vi "Dashboard Main.vi"() -> ()   [LabVIEW 2018]
uses:
  Autonomous.ctl
  <vilib>/Utility/miscctls.llb/LVRowAndColumnTypeDef.ctl
  <vilib>/event_ctls.llb/eventvkey.ctl
  <vilib>/Rock Robotics/Network Tables/NT Read Boolean.vi
  <vilib>/Rock Robotics/WPI/Dashboard/WPI_DashboardLogging Global.vi
panel:
  in  "Select Auto":T1="Select Autonomous ..."
  in  "Camera Settings Right":T2={"Frame Rate"=30, "Compression"=30, "Size"=1, "DB Camera Config"=FALSE} {"Frame Rate" scale=1.0..30.0; "Compression" scale=100.0..-1.0; "Size" items=["640x480", "320x240", "160x120"]}
  in  "Camera Name Right":string(combo)="No Camera Selection"
  out "Camera Perf":string
  in  "Camera Settings":T2={"Frame Rate"=30, "Compression"=30, "Size"=1, "DB Camera Config"=FALSE} {"Frame Rate" scale=1.0..30.0; "Compression" scale=100.0..-1.0; "Size" items=["640x480", "320x240", "160x120"]}
  in  "TCP":refnum<k5>
  in  "Rec Mode":enum32{"Stop", "Record", "Playback"}(radio)
  out "Robot IP":string
  out "Image Message":string="Timeout in Camera Communications"
  in  "Dashboard Tab":T3(tab)
  out "Cargo":bool
  out "Hatch":bool
  out "NT Connection":bool
  out "Mode":T4(ring)=enum."Auto Disabled"
  out "Right Camera Perf":cluster{"Bandwidth (Mbps)":dbl, "FPS":dbl}
  in  "Auto Selector":enum16{"Airship", "Rocket"}(ring)=enum."Rocket"
  out "Camera Image Right":T5(plugin-control)
  in  "DB/String 9":string
  in  "DB/String 8":string
  in  "DB/String 7":string
  in  "DB/String 6":string
  in  "DB/String 5":string
  in  "DB/String 4":string
  in  "DB/String 3":string
  in  "DB/String 2":string
  in  "DB/String 1":string
  in  "DB/String 0":string
  in  "DB/Slider 0":dbl(slide) scale=0.0..5.0
  in  "DB/Slider 1":dbl(slide) scale=0.0..5.0
  in  "DB/Slider 2":dbl(slide) scale=0.0..5.0
  in  "DB/Slider 3":dbl(slide) scale=0.0..5.0
  out "DB/LED 3":bool
  out "DB/LED 2":bool
  out "DB/LED 1":bool
  out "DB/LED 0":bool
  in  "DB/Button 3":bool
  in  "DB/Button 2":bool
  in  "DB/Button 1":bool
  in  "DB/Button 0":bool caption="New Name"
  out "EstadoIntake":string
  out "Yaw":dbl
  out "TracaoDir":dbl
  out "TracaoEsq":dbl
  out "Elevador Position":dbl
  out "Climber Encoder":dbl
  out "Climber State":dbl
  out "Intake Position":dbl
  in  "Test Slider":dbl(slide) scale=0.0..100.0 scale format="%#_3g"
  in  "On/Off":bool caption="Solenoid"
  in  "Test Name":u16(ring) items=["Select the test to run..."]
  in  "Test Tree":string(tree)
  in  "Motor":cluster{"Value":dbl, "Enable":bool} {"Value" scale=-1.0..1.0 scale format="%#_3g"}
  out "Progress":T6 {"Test Progress" scale=0.0..100.0}
  in  "Rev/Fwd":cluster{"Forward":bool, "Reverse":bool}
  in  "Test Ring":u16(ring) items=["Monochrome", "Color"]
  out "Cmd Status":string
  in  "Execute Command":bool
  in  "Command Params":string[][](table)
  in  "Command Selection":i32(listbox)
  in  "CheckList":i32(listbox)
  out "Tree":string(tree)
  out "Camera Image":T5(plugin-control)
  out "Background":bool
  in  "Camera Name":string(combo)="No Camera Selection"
  # "HW"
  # "HW"
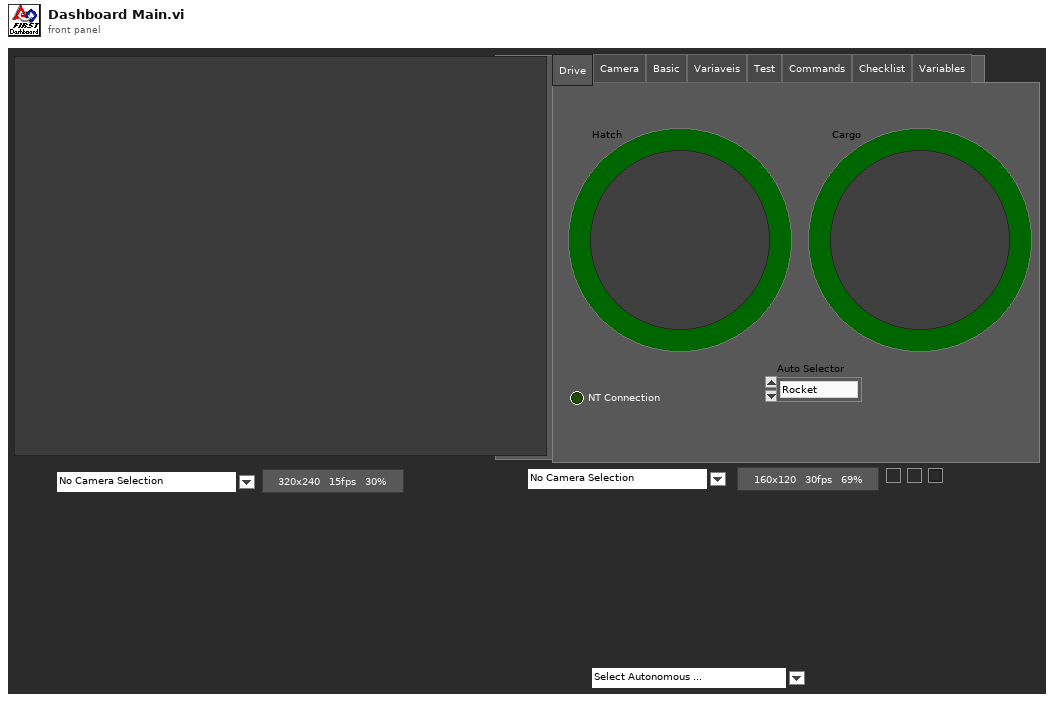
[diagram p1: front panel]
types:
  T1 = typedef "Autonomous.ctl" = string
  T2 = cluster{"Frame Rate":i32, "Compression":i32, "Size":u16, "DB Camera Config":bool}
  T3 = enum32{"Drive", "Camera", "Basic", "Variaveis", "Test", "Commands", "Checklist", "Variables"}
  T4 = enum8{"Tele-Op Disabled", "Tele-Op Enabled", "Auto Disabled", "Auto Enabled", "Test Disabled", "Test Enabled", "Disconnected", "No Code", "E-Stop"}
  T5 = typedef "IMAQ Image.ctl" = refnum<image>
  T6 = cluster{"Test Progress":u8, "Test Progress Text":string}
  T7 = cluster{"Save Path":path, "Interval (s)":dbl, "Keep":i32}
  T8 = enum32{"Drive", "Camera", "Basic", "Custom", "Test", "Commands", "Checklist", "Variables"}
  T9 = typedef "Image Type" = u32
  T10 = cluster{"IDs":cluster{"RPC field ID":u16, "Unique ID":u16}, "String":string}
  T11 = cluster{"Error Strings":string, "Disable Counts":cluster{u16, u16}, "Rail Faults":cluster{u16, u16, u16}, "Robot IP":string, "DB Mode":u8, "Event Info":cluster{"Name":string, "Type":u8, "Number":u16, "Replay":u8}}
  T12 = cluster{"Storage":cluster{"Disk Free":u64, "RAM Block":u32, "RAM free":u32}, "CPU Utilization":cluster{"CPU % ISR":sgl, "CPU % Time Crit":sgl, "CPU % Timed Str":sgl, "CPU % High":sgl, "CPU % Above":sgl, "CPU % Normal":sgl, "CPU % Low":sgl}, "CAN":cluster{"% Bus Utilization":sgl, "Bus Off Cnt":u32, "TX_FIFO Full Cnt":u32, "Receive Error Cnt":u8, "Transmit Error Cnt":u8}, "HID":cluster{"HID Outputs":u32, "Rumble Low":u16, "Rumble High":u16}[]}
  T13 = cluster{"Status bits":cluster{"Test Mode":bool, "Autonomous":bool, "Enabled":bool, "Code Start":bool, "Brownout":bool, "Reserved 2":bool, "Reserved 3":bool, "E-Stop":bool}, "Code Trace":cluster{"Disabled":bool, "TeleOp":bool, "Auto":bool, "Test":bool}, "Controller Type":enum16{"unknown", "cRIO", "roboRio"}, "Code?":enum16{"unknown", "noCode", "code"}, "Battery V":dbl}
  T14 = cluster{"Control Bits":cluster{"TestMode":bool, "Autonomous":bool, "Enabled":bool, "FMS Present":bool, bool, bool, bool, "E-Stop":bool}, "Team Station ":u8, "Countdown":sgl, "Joystick Values":cluster{"Axes":dbl[], "Buttons":bool[], "POVs":i16[]}[]}
  T15 = cluster{"Camera Image":refnum<vi>, "Dashboard Tab":refnum<vi>, "Background":refnum<vi>, "Rec Mode":refnum<vi>, "Test Slider":refnum<vi>, "On/Off ":refnum<vi>, "Test Ring":refnum<vi>, "Rev/Fwd":refnum<vi>, "Test Name":refnum<vi>, "Motor":refnum<vi>, "Progress":refnum<vi>, "CheckList":refnum<vi>, "Tree":refnum<vi>, "Test Tree":refnum<vi>, "Command Params":refnum<vi>, "Command Selection":refnum<vi>, "Execute Command":refnum<vi>, "Cmd Status":refnum<vi>, "Camera Settings":refnum<vi>, "Camera Name":refnum<vi>, "Camera Perf":refnum<vi>, "Camera Settings Right":refnum<vi>, "Camera Name Right":refnum<vi>, "Camera Image Right":refnum<vi>}
  T16 = cluster{"Global Rectangle":i32[], "Contours":cluster{"Contour Type":u32, "ROI Type":u32, "Points":i32[]}[]}
  T17 = cluster{"Camera Name":string, string, "Saved DB Images Info":cluster{"Save Path":path, "Interval (s)":dbl, "Keep":i32}}
  T18 = cluster{"Camera Name Right":string, string, "Saved DB Images Info":cluster{"Save Path":path, "Interval (s)":dbl, "Keep":i32}}
  T19 = cluster{"Operation":enum16{"Update", "Clear"}, "Color Box":u32}[]
  T20 = typedef "eventvkey.ctl" = enum16{"ASCII", "Enter", "Return", "Shift", "Ctrl", "Alt", "Cmd", "Opt", "Caps", "NumLock", "Clear", "Break", "Up", "Down", "Left", "Right", "Insert", "Delete", "Home", "End", "PageUp", "PageDown", "Escape", "Help", "Pause", "ScrollLock", "F1", "F2", "F3", "F4", "F5", "F6", "F7", "F8", "F9", "F10", "F11", "F12", "F13", "F14", "F15", "F16", "F17", "F18", "F19", "F20", "F21", "F22", "F23", "F24", "Play", "VolumeUp", "VolumeDown", "Mute", "Two Byte Char"}
  T21 = cluster{"Image Size":bool, "Image Type":bool, "Pixel Value":bool, "ROI Information":bool, "Zoom Factor":bool}
  T22 = cluster{"Operation":enum16{"Update", "Clear"}, "Color Box":u32}
  T23 = typedef "LVRowAndColumnTypeDef.ctl" = cluster{"Row":i32, "Column":i32}
  T24 = cluster{"Shift":bool, "Ctrl":bool, "Alt":bool, "Cmd":bool, "Opt":bool}
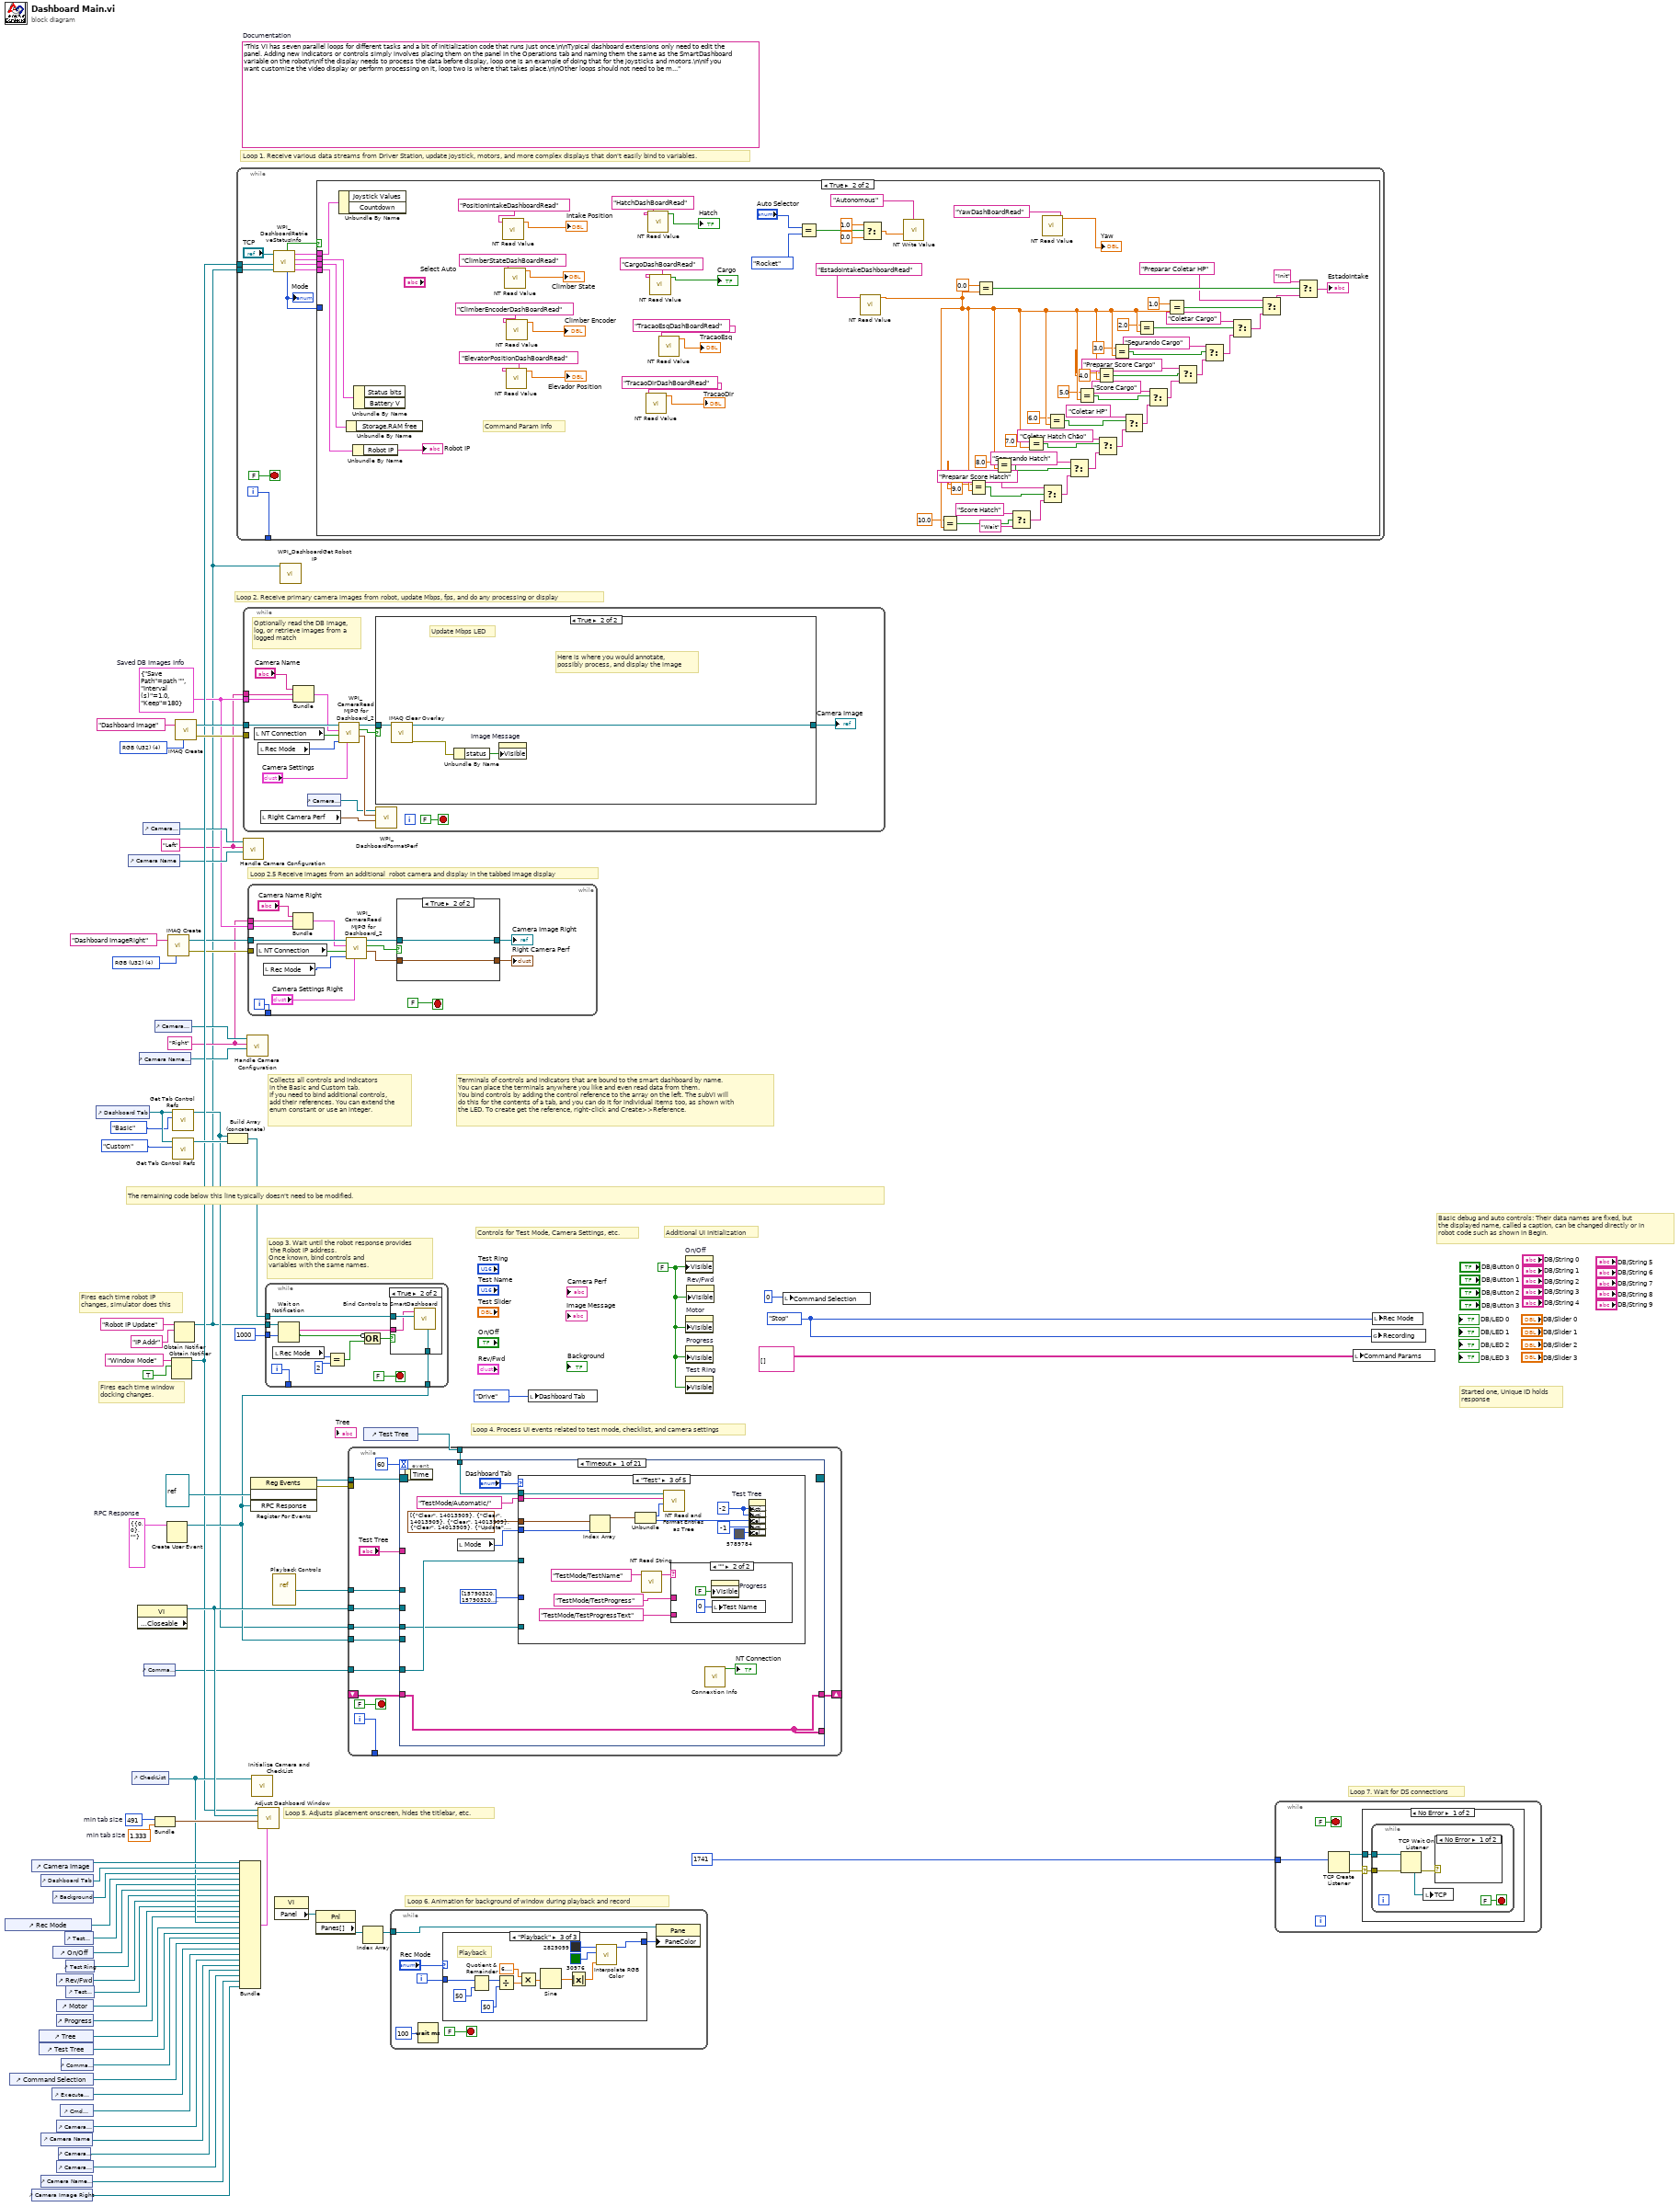
[diagram p0: block diagram]
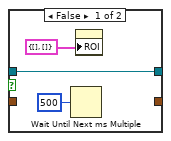
[diagram p2: hidden frame]
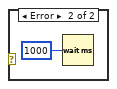
[diagram p3: hidden frame]
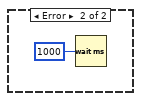
[diagram p4: hidden frame]
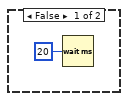
[diagram p5: hidden frame]
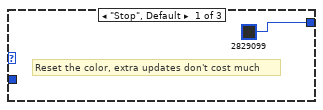
[diagram p6: hidden frame]
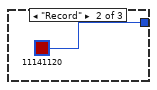
[diagram p7: hidden frame]
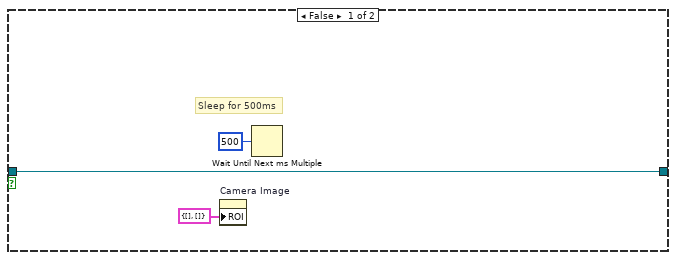
[diagram p9: hidden frame]
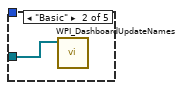
[diagram p11: hidden frame]
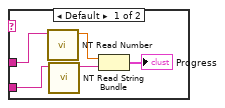
[diagram p12: hidden frame]
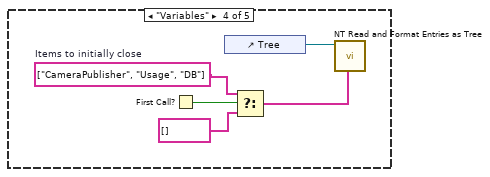
[diagram p13: hidden frame]
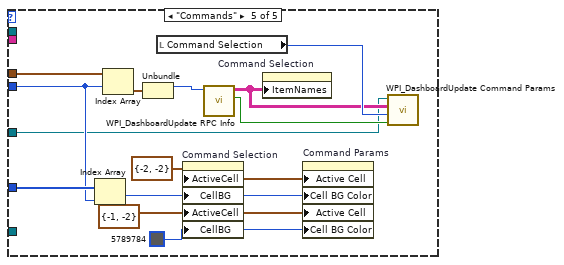
[diagram p14: hidden frame]
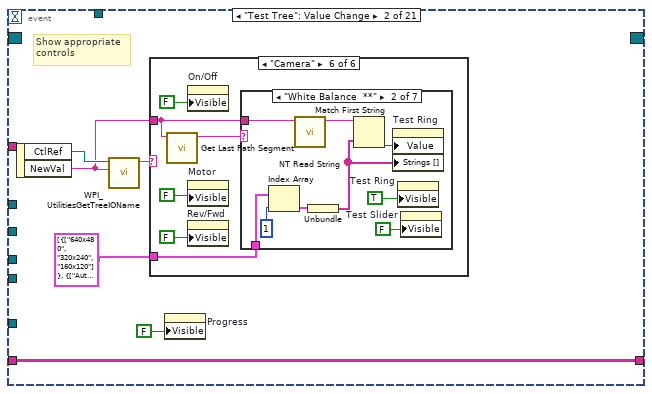
[diagram p15: hidden frame]
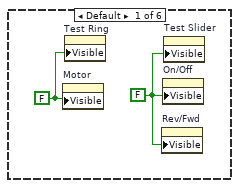
[diagram p16: hidden frame]
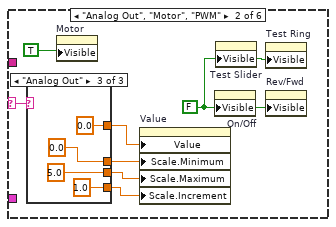
[diagram p17: hidden frame]
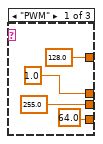
[diagram p18: hidden frame]
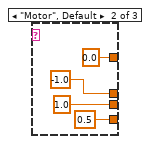
[diagram p19: hidden frame]
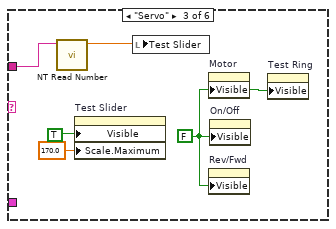
[diagram p20: hidden frame]
diagram:
  w4 = T7 {"Save Path"=path "", "Interval (s)"=1.0, "Keep"=180}  # Saved DB Images Info
  w3 = "Right"
  w2 = "Left"
  w14 = T9 4 items=["Grayscale (U8)", "Grayscale (I16)", "Grayscale (SGL)", "Complex (CSG)", "RGB (U32)", "HSL (U32)", "RGB (U64)"] ("Image Type")
  w28 = T10 {"IDs"={"RPC field ID"=0, "Unique ID"=0}, "String"=""}  # RPC Response
  w50 = 491  # min tab size
  w49 = 1.333  # min tab size
  w57 = enum32{"Stop", "Record", "Playback"}."Stop" ("Rec Mode")
  w34 = FALSE ("Visible")
  (unwired) "This VI has seven parallel loops for different tasks and a bit of initialization code that runs just once.\n\nTypical dashboard extensions only need to edit the panel. Adding new indicators or controls simply involves placing them on the panel in the Operations tab and naming them the same as the SmartDashboard variable on the robot\n\nIf the display needs to process the data before display, loop one is an example of doing that for the joysticks and motors.\n\nIf you want customize the video display or perform processing on it, loop two is where that takes place.\n\nOther loops should not need to be modified. They are pretty standard, and document the task they perform."  # Documentation
  w74 = T9 4 items=["Grayscale (U8)", "Grayscale (I16)", "Grayscale (SGL)", "Complex (CSG)", "RGB (U32)", "HSL (U32)", "RGB (U64)"] ("Image Type")
  # "Loop 2.5 Receive images from an additional  robot camera and display in the tabbed image display"
  # "Started one, Unique ID holds\nresponse"
  # "Loop 7. Wait for DS connections"
  # "Basic debug and auto controls: Their data names are fixed, but\nthe displayed name, called a caption, can be changed directly or in\nrobot code such as shown in Begin."
  # "Controls for Test Mode, Camera Settings, etc."
  # "Additional UI Initialization"
  # "Loop 6. Animation for background of window during playback and record"
  # "Fires each time robot IP\nchanges, simulator does this"
  # "Fires each time window\ndocking changes."
  # "Collects all controls and indicators\nin the Basic and Custom tab.\nIf you need to bind additional controls,\nadd their references. You can extend the\nenum constant or use an integer."
  # "The remaining code below this line typically doesn't need to be modified."
  # "Loop 4. Process UI events related to test mode, checklist, and camera settings"
  # "Terminals of controls and indicators that are bound to the smart dashboard by name.\nYou can place the terminals anywhere you like and even read data from them.\nYou bind controls by adding the control reference to the array on the left. The subVI will\ndo this for the contents of a tab, and you can do it for individual items too, as shown with\nthe LED. To create get the reference, right-click and Create>>Reference."
  # "Loop 3. Wait until the robot response provides\n the Robot IP address.\nOnce known, bind controls and\nvariables with the same names."
  # "Loop 5. Adjusts placement onscreen, hides the titlebar, etc."
  # "Loop 1. Receive various data streams from Driver Station, update joystick, motors, and more complex displays that don't easily bind to variables."
  # "Loop 2. Receive primary camera images from robot, update Mbps, fps, and do any processing or display"
  n1 = control-ref of="Rec Mode"() -> (w40:refnum<vi>)
  n2 = control-ref of="Command Selection"() -> (w27:refnum<vi>)
  n3 = control-ref of="Camera Image Right"() -> (w7:refnum<vi>)
  n4 = control-ref of="Camera Image"() -> (w52:refnum<vi>)
  n5 = control-ref of="Tree"() -> (w44:refnum<vi>)
  n6 = control-ref of="Test Tree"() -> (w43:refnum<vi>)
  n7 = control-ref of="Dashboard Tab"() -> (w51:refnum<vi>)
  n8 = control-ref of="Camera Name"() -> (w18:refnum<vi>)
  n9 = control-ref of="Camera Name Right"() -> (w8:refnum<vi>)
  n10 = control-ref of="Execute Command"() -> (w29:refnum<vi>)
  n11 = control-ref of="Background"() -> (w47:refnum<vi>)
  n12 = control-ref of="On/Off"() -> (w38:refnum<vi>)
  n13 = control-ref of="Progress"() -> (w35:refnum<vi>)
  n14 = control-ref of="Camera Settings"() -> (w19:refnum<vi>)
  n15 = control-ref of="Camera Settings Right"() -> (w9:refnum<vi>)
  n16 = control-ref of="Rev/Fwd"() -> (w36:refnum<vi>)
  n17 = control-ref of="Motor"() -> (w41:refnum<vi>)
  n18 = control-ref of="Camera Perf"() -> (w17:refnum<vi>)
  n19 = control-ref of="Cmd Status"() -> (w23:refnum<vi>)
  n20 = control-ref of="Command Params"() -> (w30:refnum<vi>)
  n21 = control-ref of="Test Slider"() -> (w39:refnum<vi>)
  n22 = control-ref of="Test Ring"() -> (w37:refnum<vi>)
  n23 = control-ref of="Test Name"() -> (w42:refnum<vi>)
  n24 = control-ref of="Dashboard Tab"() -> (w55:refnum<vi>)
  n25 = control-ref of="Camera Name"() -> (w20:refnum<vi>)
  n26 = control-ref of="CheckList"() -> (w45:refnum<vi>)
  n27 = property class="VI" props=["Front Panel.Closeable"]() -> (reference out=w56:refnum<vi>)  [unwired: 2 in, 2 out]
  n28 = control-ref of="Camera Name Right"() -> (w10:refnum<vi>)
  n29 = control-ref of="Camera Settings"() -> (w21:refnum<vi>)
  n30 = control-ref of="Command Params"() -> (w22:refnum<vi>)
  n31 = control-ref of="Camera Settings Right"() -> (w11:refnum<vi>)
  n32 = Bundle("min tab size"=w50, "min tab size"=w49) -> (w48:cluster{"min tab size":i32, "min tab size":dbl})  [unwired: 1 in]
  n33 = Create User Event(user event datatype=w28) -> (user event=w24:refnum<user-event>)  [unwired: 1 in, 1 out]
  n34 = call "IMAQ Create"("Image Name"="Dashboard ImageRight", "Image Type"=w14) -> ("New Image"=w13:T5, "error out"=w12:errorcluster)  [unwired: 2 in, 1 out]
  n35 = Obtain Notifier(name (unnamed)="Window Mode", notification data type=TRUE) -> (notifier out=w33:refnum<notifier>)  [unwired: 2 in, 2 out]
  n36 = call <vilib>:"Get Tab Control Refs.vi"("Page Index"=T8."Basic" ("Dashboard Tab"), "TabControl in"=w55) -> ("ControlsOnPage"=w16:refnum<vi>[])  [unwired: 9 in]
  n37 = call <vilib>:"Get Tab Control Refs.vi"("Page Index"=T8."Custom" ("Dashboard Tab"), "TabControl in"=w55) -> ("ControlsOnPage"=w54:refnum<vi>[])  [unwired: 9 in]
  n38 = Obtain Notifier(name (unnamed)="Robot IP Update", notification data type="IP Addr" ("name (unnamed)")) -> (notifier out=w1:refnum<notifier>)  [unwired: 2 in, 2 out]
  n39 = call "IMAQ Create"("Image Name"="Dashboard Image", "Image Type"=w74) -> ("New Image"=w72:T5, "error out"=w71:errorcluster)  [unwired: 2 in, 1 out]
  n40 = Build Array (concatenate)(w16, w54) -> (w53:refnum<vi>[])
  n41 = while {
    tunnel: [w84] -> _
    tunnel: w1 -> [w78]
    tunnel: w33 -> [w75]
    i -> [w84]
    stop <- FALSE stop-if-true
    n42 = call <vilib>:"WPI_DashboardRetrieveStatusInfo.vi"("Binding Refnum"=w78, "Window Mode Notifier"=w75, "TCP Cnx"="TCP") -> ("Power and Errors"=w79:T11, "Robot Metrics"=w82:T12, "Status Info"=w83:T13, "Control Info"=w80:T14, "Robot Mode"=w77:T4, "Process?"=w81:bool)  [unwired: 3 in]
    "Mode" <- w77
    n43 = case shown="True" w81 {
      tunnel: w83 -> [_ w163]
      tunnel: w82 -> [_ w162]
      tunnel: w80 -> [_ w161]
      tunnel: w79 -> [_ w160]
      tunnel: w77 -> [_ _]
      frame False {
        n44 = Wait (ms)(milliseconds to wait=u32 20) -> ()  [unwired: 1 out]
      }
      frame True {
        # "Command Param Info"
        n45 = Unbundle By Name(w161) -> ()  [unwired: 2 out]
        n46 = Unbundle By Name(w162) -> ()  [unwired: 1 out]
        n47 = Unbundle By Name(w160) -> ("Robot IP"=→"Robot IP":string)
        n48 = Unbundle By Name(w163) -> ()  [unwired: 2 out]
        n49 = call-poly <vilib>:"NT Read Value.vi"("Name"="PositionIntakeDashboardRead") -> ("Numeric"=→"Intake Position":dbl)  [unwired: 9 in, 1 out]
        n50 = call-poly <vilib>:"NT Read Value.vi"("Name"="ClimberStateDashBoardRead") -> ("Numeric"=→"Climber State":dbl)  [unwired: 9 in, 1 out]
        n51 = call-poly <vilib>:"NT Read Value.vi"("Name"="ElevatorPositionDashBoardRead") -> ("Numeric"=→"Elevador Position":dbl)  [unwired: 9 in, 1 out]
        n52 = call-poly <vilib>:"NT Read Value.vi"("Name"="ClimberEncoderDashBoardRead") -> ("Numeric"=→"Climber Encoder":dbl)  [unwired: 9 in, 1 out]
        n53 = call-poly <vilib>:"NT Read Value.vi"("Name"="TracaoDirDashBoardRead") -> ("Numeric"=→"TracaoDir":dbl)  [unwired: 9 in, 1 out]
        n54 = call-poly <vilib>:"NT Read Value.vi"("Name"="HatchDashBoardRead") -> ("Boolean"=→"Hatch":bool)  [unwired: 9 in, 1 out]
        n55 = call-poly <vilib>:"NT Read Value.vi"("Name"="CargoDashBoardRead") -> ("Boolean"=→"Cargo":bool)  [unwired: 9 in, 1 out]
        n56 = call-poly <vilib>:"NT Read Value.vi"("Name"="TracaoEsqDashBoardRead") -> ("Numeric"=→"TracaoEsq":dbl)  [unwired: 9 in, 1 out]
        n57 = Equal?(x="Auto Selector", y=enum16{"Airship", "Rocket"}."Rocket") -> (x = y?=w141:bool)
        n58 = call-poly <vilib>:"NT Read Value.vi"("Name"="EstadoIntakeDashboardRead") -> ("Numeric"=w135:dbl)  [unwired: 9 in, 1 out]
        n59 = Select(t=1.0, s=w141, f=0.0) -> (s? t:f=w142:dbl)
        n60 = call-poly <vilib>:"NT Write Value.vi"("Numeric"=w142, "Name"="Autonomous") -> ()  [unwired: 9 in, 1 out]
        n61 = Equal?(x=10.0, y=w135) -> (x = y?=w134:bool)
        n62 = Equal?(x=9.0, y=w135) -> (x = y?=w133:bool)
        n63 = Equal?(x=0.0, y=w135) -> (x = y?=w113:bool)
        n64 = Equal?(x=8.0, y=w135) -> (x = y?=w132:bool)
        n65 = Select(t="Score Hatch", s=w134, f="Wait") -> (s? t:f=w126:string)
        n66 = Equal?(x=7.0, y=w135) -> (x = y?=w131:bool)
        n67 = call-poly <vilib>:"NT Read Value.vi"("Name"="YawDashBoardRead") -> ("Numeric"=→"Yaw":dbl)  [unwired: 9 in, 1 out]
        n68 = Select(t="Preparar Score Hatch", s=w133, f=w126) -> (s? t:f=w125:string)
        n69 = Equal?(x=6.0, y=w135) -> (x = y?=w130:bool)
        n70 = Select(t="Segurando Hatch", s=w132, f=w125) -> (s? t:f=w124:string)
        n71 = Equal?(x=5.0, y=w135) -> (x = y?=w129:bool)
        n72 = Equal?(x=4.0, y=w135) -> (x = y?=w128:bool)
        n73 = Select(t="Coletar Hatch Chão", s=w131, f=w124) -> (s? t:f=w123:string)
        n74 = Equal?(x=3.0, y=w135) -> (x = y?=w127:bool)
        n75 = Select(t="Coletar HP", s=w130, f=w123) -> (s? t:f=w122:string)
        n76 = Equal?(x=2.0, y=w135) -> (x = y?=w117:bool)
        n77 = Select(t="Score Cargo", s=w129, f=w122) -> (s? t:f=w121:string)
        n78 = Equal?(x=1.0, y=w135) -> (x = y?=w116:bool)
        n79 = Select(t="Preparar Score Cargo", s=w128, f=w121) -> (s? t:f=w120:string)
        n80 = Select(t="Segurando Cargo", s=w127, f=w120) -> (s? t:f=w119:string)
        n81 = Select(t="Coletar Cargo", s=w117, f=w119) -> (s? t:f=w118:string)
        n82 = Select(t="Preparar Coletar HP", s=w116, f=w118) -> (s? t:f=w115:string)
        n83 = Select(t="Init", s=w113, f=w115) -> (s? t:f=→"EstadoIntake":string)
      }
    }
  }
  n84 = Bundle("Camera Image"=w52, "Dashboard Tab"=w51, "Background"=w47, "Rec Mode"=w40, "Test Slider"=w39, "On/Off"=w38, "Test Ring"=w37, "Rev/Fwd"=w36, "Test Name"=w42, "Motor"=w41, "Progress"=w35, "CheckList"=w45, "Tree"=w44, "Test Tree"=w43, "Command Params"=w30, "Command Selection"=w27, "Execute Command"=w29, "Cmd Status"=w23, "Camera Settings"=w19, "Camera Name"=w18, "Camera Perf"=w17, "Camera Settings Right"=w9, "Camera Name Right"=w8, "Camera Image Right"=w7) -> (w46:T15)  [unwired: 1 in]
  n85 = call "Handle Camera Configuration.vi"("CameraNameRef"=w20, "Display Name"=w2, "ClusterRef"=w21) -> ()  [unwired: 9 in]
  n86 = while {
    tunnel: w72 -> [w177]
    tunnel: w71 -> [_]
    tunnel: w4 -> [w170]
    tunnel: w2 -> [w167]
    stop <- FALSE stop-if-true
    # "Optionally read the DB image,\nlog, or retrieve images from a\nlogged match"
    n87 = local read "NT Connection"() -> (w171:bool)
    n88 = local read "Rec Mode"() -> (w174:enum32{"Stop", "Record", "Playback"})
    n89 = local read "Right Camera Perf"() -> (w165:cluster{"Bandwidth (Mbps)":dbl, "FPS":dbl})
    n90 = Bundle("Camera Name"="Camera Name", w167, "Saved DB Images Info"=w170) -> (w169:T17)  [unwired: 1 in]
    n91 = control-ref of="Camera Perf"() -> (w164:refnum<vi>)
    n92 = call <vilib>:"WPI_CameraRead MJPG for Dashboard_2.vi"("Camera Settings"="Camera Settings", "Rec Mode"=w174, "NT Connection"=w171, "Capture Info"=w169, "Image in"=w177) -> ("perf info"=w166:cluster{"Bandwidth (Mbps)":dbl, "fps":dbl}, "Active"=w175:bool, "Image\\ out"=w176:T5)  [unwired: 4 in]
    n93 = case shown="True" w175 {
      tunnel: w176 -> [w180 w183]
      tunnel: [w180 w182] -> w172
      frame False {
        # "Sleep for 500ms"
        n94 = property on="Camera Image" class="ImageControl"("ROI"=T16 {"Global Rectangle"=[], "Contours"=[]}) -> ()  [unwired: 2 in, 2 out]
        n95 = Wait Until Next ms Multiple(millisecond multiple=u32 500) -> ()  [unwired: 1 out]
      }
      frame True {
        # "Here is where you would annotate,\npossibly process, and display the image"
        # "Update Mbps LED"
        n96 = call "IMAQ Clear Overlay"("Image"=w183) -> ("error out"=w184:errorcluster, "Image Out"=w182:T5)  [unwired: 2 in, 7 out]
        n97 = Unbundle By Name(w184) -> ("status"=w185:bool)
        n98 = property on="Image Message" class="Str"("Visible"=w185) -> ()  [unwired: 2 in, 2 out]
      }
    }
    "Camera Image" <- w172
    n99 = call <vilib>:"WPI_DashboardFormatPerf.vi"("Right Camera Perf"=w165, "Performance"=w166, "String in"=w164) -> ()  [unwired: 9 in]
  }
  n100 = call "Handle Camera Configuration.vi"("CameraNameRef"=w10, "Display Name"=w3, "ClusterRef"=w11) -> ()  [unwired: 9 in]
  n101 = while {
    tunnel: w13 -> [w200]
    tunnel: w12 -> [_]
    tunnel: [w195] -> _
    tunnel: w4 -> [w191]
    tunnel: w3 -> [w188]
    i -> [w195]
    stop <- FALSE stop-if-true
    n102 = local read "NT Connection"() -> (w192:bool)
    n103 = local read "Rec Mode"() -> (w199:enum32{"Stop", "Record", "Playback"})
    n104 = Bundle("Camera Name Right"="Camera Name Right", w188, "Saved DB Images Info"=w191) -> (w190:T18)  [unwired: 1 in]
    n105 = call <vilib>:"WPI_CameraRead MJPG for Dashboard_2.vi"("Camera Settings"="Camera Settings Right", "Rec Mode"=w199, "NT Connection"=w192, "Capture Info"=w190, "Image in"=w200) -> ("perf info"=w186:cluster{"Bandwidth (Mbps)":dbl, "fps":dbl}, "Active"=w194:bool, "Image\\ out"=w197:T5)  [unwired: 4 in]
    n106 = case shown="True" w194 {
      tunnel: w197 -> [w202 w205]
      tunnel: [w202 w205] -> w193
      tunnel: [_ w204] -> w187
      tunnel: w186 -> [_ w204]
      frame False {
        n107 = Wait Until Next ms Multiple(millisecond multiple=u32 500) -> ()  [unwired: 1 out]
        n108 = property on="Camera Image Right" class="ImageControl"("ROI"=T16 {"Global Rectangle"=[], "Contours"=[]}) -> ()  [unwired: 2 in, 2 out]
      }
      frame True {
      }
    }
    "Camera Image Right" <- w193
    "Right Camera Perf" <- w187
  }
  n109 = register-events(refnum<vi> refnum, w24) -> (reference out=w61:refnum<event-registration>, error out=w60:errorcluster)  [unwired: 2 in]
  n110 = call "Initialize Camera and CheckList.vi"("ListBox in"=w45) -> ()  [unwired: 11 in]
  n111 = call "Adjust Dashboard Window.vi"("Sizing Refnums"=w46, "Size Constraints"=w48, "VI"=w56, "WIn Mode"=w33) -> ()  [unwired: 8 in]
  n112 = while {
    tunnel: w53 -> [w217]
    tunnel: w1 -> [w215]
    tunnel: [w213] -> _
    tunnel: u32 1000 ("milliseconds to wait") -> [w212]
    tunnel: w24 -> [w206]
    i -> [w213]
    stop <- FALSE stop-if-true
    n113 = local read "Rec Mode"() -> (w208:enum32{"Stop", "Record", "Playback"})
    n114 = Wait on Notification(notifier=w215, timeout in ms (-1)=w212) -> (notification=w214:string, timed out?=w210:bool)  [unwired: 2 in, 2 out]
    n115 = Equal?(x=w208, y=u16 2 ("Rec Mode")) -> (x = y?=w209:bool)
    n116 = Compound Arithmetic op=OR(invert w210, w209) -> (w211:bool)
    n117 = case shown="True" w211 {
      tunnel: w217 -> [_ w220]
      tunnel: w214 -> [_ w219]
      tunnel: w206 -> [_ w218]
      frame False {
      }
      frame True {
        n118 = call <vilib>:"Bind Controls to SmartDashboard.vi"("RPC ref"=w218, "Bound Control Refs"=w220, "Server IP Address"=w219) -> ()  [unwired: 9 in]
      }
    }
  }
  n119 = vi-ref "Playback Controls.vi"() -> (w62:refnum<vi>)
  n120 = property class="VI"() -> ("Panel"=w64:refnum<vi>)  [unwired: 2 in, 2 out]
  n121 = call "WPI_DashboardGet Robot IP.vi"("Notifier in"=w1) -> ()  [unwired: 11 in]
  n122 = property class="Pnl"(reference=w64) -> ("Panes[]"=w65:refnum<vi>[])  [unwired: 1 in, 2 out]
  n123 = Index Array(array=w65) -> (element=w63:refnum<vi>)  [unwired: 1 in]
  n124 = control-ref of="Test Tree"() -> (w66:refnum<vi>)
  n125 = while {
    tunnel: [w230] -> _
    tunnel: w66 -> [w229]
    tunnel: w62 -> [w228]
    tunnel: w61 -> [w227]
    tunnel: w60 -> [_]
    tunnel: w56 -> [w226]
    tunnel: w24 -> [w225]
    tunnel: w22 -> [w224]
    shift-right: [w223] -> _
    shift-left: _ -> [w222]
    tunnel: w16 -> [w221]
    i -> [w230]
    stop <- FALSE stop-if-true
    n126 = event shown="[0] Timeout" {
      selector: w227 -> [_ _ _ _ _ _ _ _ _ _ _ _ _ _ _ _ _ _ _ _ _]
      dyn-events: [_ _ _ _ _ _ _ _ _ _ _ _ _ _ _ _ w490 _ _ _ _] -> _
      timeout: u32 60 ("milliseconds to wait") -> [_ _ _ _ _ _ _ _ _ _ _ _ _ _ _ _ _ _ _ _ _]
      tunnel: w229 -> [w242 _ _ _ _ _ _ _ _ _ _ _ _ _ _ _ _ _ _ _ _]
      tunnel: "Test Tree" -> [_ _ _ _ _ _ _ _ _ _ _ w457 w465 w467 w471 w479 _ _ _ _ _]
      tunnel: w228 -> [_ _ _ _ _ _ _ _ _ _ _ _ _ _ _ _ w492 _ w510 _ _]
      tunnel: w226 -> [_ _ _ _ _ _ _ _ _ _ _ _ _ _ _ _ w488 _ _ _ _]
      tunnel: w225 -> [_ _ _ _ _ _ _ _ _ _ _ _ _ _ _ _ w486 _ _ _ _]
      tunnel: w224 -> [w237 _ _ _ _ _ w408 _ _ _ _ _ _ _ _ _ _ _ _ _ _]
      tunnel: [w234 w285 w387 w392 w401 w405 w406 w415 w425 w432 w444 w456 w463 w466 w470 w478 w485 w505 w507 w511 w524] -> w223
      tunnel: w222 -> [w234 w285 w387 w392 w401 w405 w406 _ _ w432 w444 w456 w463 w466 w470 w478 w485 w505 w507 w511 w524]
      tunnel: w221 -> [w235 _ _ _ _ _ _ _ _ _ _ _ _ _ _ _ _ _ _ _ _]
      tunnel: [w234 _ _ _ _ _ _ _ _ _ _ _ _ _ _ _ _ _ _ _ _] -> _
      event Timeout {
        n127 = event-data() -> ()  [unwired: 1 in, 1 out]
        n128 = local read "Mode"() -> (w239:T4)
        n129 = case shown="\"Test\"" "Dashboard Tab" {
          tunnel: w242 -> [_ _ w258 _ _]
          tunnel: "TestMode/Automatic/" ("Name Pattern") -> [_ _ w257 _ _]
          tunnel: T19 [{"Operation"=enum."Clear", "Color Box"=14013909}, {"Operation"=enum."Clear", "Color Box"=14013909}, {"Operation"=enum."Clear", "Color Box"=14013909}, {"Operation"=enum."Clear", "Color Box"=14013909}, {"Operation"=enum."Update", "Color Box"=14013909}, {"Operation"=enum."Update", "Color Box"=16777215}, {"Operation"=enum."Clear", "Color Box"=14013909}, {"Operation"=enum."Clear", "Color Box"=14013909}, {"Operation"=enum."Clear", "Color Box"=14013909}] -> [_ _ w250 _ w278]
          tunnel: w239 -> [_ _ w249 _ w277]
          tunnel: u32[] [15790320, 15790320, 15790320, 15790320, 16777215, 16777215, 15790320, 15790320, 15790320] -> [_ _ _ _ w283]
          tunnel: w237 -> [_ _ _ _ w271]
          tunnel: w235 -> [_ w244 _ _ _]
          frame "Variaveis", Default {
          }
          frame "Basic" {
            n130 = call <vilib>:"WPI_DashboardUpdateNames.vi"("Controls on Tab"=w244) -> ()  [unwired: 11 in]
          }
          frame "Test" {
            w256 = -2 ("Active Item:Row Number")
            n131 = Index Array(array=w250, index=w249) -> (element=w251:T22)
            n132 = Unbundle(w251) -> ("Operation"=w252:enum16{"Update", "Clear"}, "Color Box"=w253:u32)
            n133 = call <vilib>:"NT Read String.vi"("Name"="TestMode/TestName") -> ("String"=w247:string)  [unwired: 9 in, 1 out]
            n134 = call <vilib>:"NT Read and Format Entries as Tree.vi"("Operation"=w252, "Name Pattern"=w257, "Tree Refnum"=w258) -> ()  [unwired: 7 in, 2 out]
            n135 = case shown="\"\"" w247 {
              tunnel: "TestMode/TestProgress" ("Name") -> [w260 _]
              tunnel: "TestMode/TestProgressText" ("Name") -> [w259 _]
              frame Default {
                n136 = call <vilib>:"NT Read Number.vi"("Name"=w260) -> ("Numeric"=w261:dbl)  [unwired: 9 in, 1 out]
                n137 = call <vilib>:"NT Read String.vi"("Name"=w259) -> ("String"=w262:string)  [unwired: 9 in, 1 out]
                n138 = Bundle("Numeric"=w261, "String"=w262) -> (→"Progress":cluster{"Numeric":dbl, "String":string})  [unwired: 1 in]
              }
              frame "" {
                n139 = property on="Progress" class="Clust (strict)"("Visible"=FALSE) -> ()  [unwired: 2 in, 2 out]
                n140 = local write "Test Name"(u16 0) -> ()
              }
            }
            n141 = property on="Test Tree" class="Tree (strict)"("Active Item Row Number"=w256, "ActiveColNum"=w256, "CellBG"=w253, "Active Item Row Number"=-1 ("Active Item:Row Number"), "CellBG"=u32 5789784 ("Color Box")) -> ()  [unwired: 2 in, 2 out]
          }
          frame "Variables" {
            w268 = string[] ["CameraPublisher", "Usage", "DB"]  # Items to initially close
            n142 = First Call?() -> (First Call?: T/F=w269:bool)
            n143 = control-ref of="Tree"() -> (w270:refnum<vi>)
            n144 = Select(t=w268, s=w269, f=string[] []) -> (s? t:f=w266:string[])
            n145 = call <vilib>:"NT Read and Format Entries as Tree.vi"("Tags to  Close"=w266, "Tree Refnum"=w270) -> ()  [unwired: 8 in, 2 out]
          }
          frame "Commands" {
            w279 = u32 5789784 ("Color Box")
            w280 = T23 {"Row"=-1, "Column"=-2} ("Active Cell:Active Cell")
            w282 = T23 {"Row"=-2, "Column"=-2} ("Active Cell:Active Cell")
            n146 = Index Array(array=w283, index=w277) -> (element=w281:u32)
            n147 = Index Array(array=w278, index=w277) -> (element=w276:T22)
            n148 = Unbundle(w276) -> ("Operation"=w275:enum16{"Update", "Clear"})  [unwired: 1 out]
            n149 = local read "Command Selection"() -> (w274:i32)
            n150 = property on="Command Selection" class="MCListbox (strict)"("ActiveCell"=w282, "CellBG"=w281, "ActiveCell"=w280, "CellBG"=w279) -> ()  [unwired: 2 in, 2 out]
            n151 = call <vilib>:"WPI_DashboardUpdate RPC Info.vi"("Operation"=w275) -> ("update"=w273:bool, "commands"=w272:string[][])  [unwired: 9 in]
            n152 = property on="Command Selection" class="MCListbox (strict)"("ItemNames"=w272) -> ()  [unwired: 2 in, 2 out]
            n153 = property on="Command Params" class="Tbl (strict)"("Active Cell"=w282, "Cell BG Color"=w281, "Active Cell"=w280, "Cell BG Color"=w279) -> ()  [unwired: 2 in, 2 out]
            n154 = call <vilib>:"WPI_DashboardUpdate Command Params.vi"("Update"=w273, "NewVal"=w274, "Commands"=w272, "Param Tbl"=w271) -> ()  [unwired: 7 in, 1 out]
          }
        }
        n155 = call <vilib>:"Connextion Info.vi"() -> ("Connected"=→"NT Connection":bool)  [unwired: 10 in, 1 out]
      }
      event "Test Tree": Value Change {
        # "Show appropriate\ncontrols"
        n156 = event-data() -> ("CtlRef"=w288:refnum<vi>, "NewVal"=w286:string)  [unwired: 1 in]
        n157 = call <vilib>:"WPI_UtilitiesGetTreeIOName.vi"("NewVal"=w286, "TreeControl in"=w288) -> ("I/O Name"=w289:string)  [unwired: 9 in]
        n158 = case shown="\"Camera\"" w289 {
          selector: w289 -> [_ w296 _ w318 w327 _]
          tunnel: w286 -> [_ _ w315 w317 _ w334]
          tunnel: cluster{string[]}[] [{["640x480", "320x240", "160x120"]}, {["Auto", "Fixed indoor", "Fixed outdoor 1", "Fixed outdoor 2", "Fixed fluorescent 1", "Fixed fluorescent 2", "Hold current"]}, {["Auto", "Flicker-free 50 Hz", "Flicker-free 60 Hz", "Hold current"]}, {["None", "Prioritize frame rate", "Prioritize image quality"]}, {["Monochrome", "Color"]}] -> [_ _ _ _ _ w333]
          frame Default {
            w291 = FALSE ("Visible")
            w290 = FALSE ("Visible")
            n159 = property on="Motor" class="Clust (strict)"("Visible"=w290) -> ()  [unwired: 2 in, 2 out]
            n160 = property on="Test Ring" class="Ring (strict)"("Visible"=w290) -> ()  [unwired: 2 in, 2 out]
            n161 = property on="Rev/Fwd" class="Clust (strict)"("Visible"=w291) -> ()  [unwired: 2 in, 2 out]
            n162 = property on="On/Off" class="Bool (strict)"("Visible"=w291) -> ()  [unwired: 2 in, 2 out]
            n163 = property on="Test Slider" class="Slide (strict)"("Visible"=w291) -> ()  [unwired: 2 in, 2 out]
          }
          frame "Analog Out", "Motor", "PWM" {
            w297 = FALSE ("Visible")
            n164 = case shown="\"Analog Out\"" w296 {
              tunnel: [1.0 ("Value") -1.0 ("Value") 0.0 ("Value")] -> w295
              tunnel: [255.0 ("Value") 1.0 ("Value") 5.0 ("Value")] -> w294
              tunnel: [128.0 ("Value") 0.0 ("Value") 0.0 ("Value")] -> w293
              tunnel: [64.0 ("Value") 0.5 ("Value") 1.0 ("Value")] -> w292
              frame "PWM" {
              }
              frame "Motor", Default {
              }
              frame "Analog Out" {
              }
            }
            n165 = property on="Motor" class="Clust (strict)"("Visible"=TRUE) -> ()  [unwired: 2 in, 2 out]
            n166 = property on="Value" class="Slide (strict)"("Value"=w293, "Scale.Minimum"=w295, "Scale.Maximum"=w294, "Scale.Increment"=w292) -> ()  [unwired: 2 in, 2 out]
            n167 = property on="On/Off" class="Bool (strict)"("Visible"=w297) -> ()  [unwired: 2 in, 2 out]
            n168 = property on="Test Slider" class="Slide (strict)"("Visible"=w297) -> ()  [unwired: 2 in, 2 out]
            n169 = property on="Test Ring" class="Ring (strict)"("Visible"=w297) -> ()  [unwired: 2 in, 2 out]
            n170 = property on="Rev/Fwd" class="Clust (strict)"("Visible"=w297) -> ()  [unwired: 2 in, 2 out]
          }
          frame "Servo" {
            w313 = FALSE ("Visible")
            n171 = call <vilib>:"NT Read Number.vi"("Name"=w315) -> ("Numeric"=w314:dbl)  [unwired: 9 in, 1 out]
            n172 = property on="Test Slider" class="Slide (strict)"("Visible"=TRUE, "Scale.Maximum"=170.0 ("Scale.Range:Maximum")) -> ()  [unwired: 2 in, 2 out]
            n173 = local write "Test Slider"(w314) -> ()
            n174 = property on="Motor" class="Clust (strict)"("Visible"=w313) -> ()  [unwired: 2 in, 2 out]
            n175 = property on="Rev/Fwd" class="Clust (strict)"("Visible"=w313) -> ()  [unwired: 2 in, 2 out]
            n176 = property on="On/Off" class="Bool (strict)"("Visible"=w313) -> ()  [unwired: 2 in, 2 out]
            n177 = property on="Test Ring" class="Ring (strict)"("Visible"=w313) -> ()  [unwired: 2 in, 2 out]
          }
          frame "Relay", "Solenoid" {
            w316 = FALSE ("Visible")
            n178 = property on="Motor" class="Clust (strict)"("Visible"=w316) -> ()  [unwired: 2 in, 2 out]
            n179 = property on="Test Slider" class="Slide (strict)"("Visible"=w316) -> ()  [unwired: 2 in, 2 out]
            n180 = Search and Replace String(input string=w317, search string="/Value  **", replace string="/Direction") -> (result string=w323:string)  [unwired: 5 in, 3 out]
            n181 = property on="Test Ring" class="Ring (strict)"("Visible"=w316) -> ()  [unwired: 2 in, 2 out]
            n182 = call <vilib>:"NT Read String.vi"("Name"=w323) -> ("String"=w321:string)  [unwired: 9 in, 1 out]
            n183 = Equal?(x="Both directions", y=w321) -> (x = y?=w319:bool)
            n184 = Not(x=w319) -> (.not. x?=w320:bool)
            n185 = property on="Rev/Fwd" class="Clust (strict)"("Visible"=w319) -> ()  [unwired: 2 in, 2 out]
            n186 = property on="On/Off" class="Bool (strict)"("Visible"=w320, "Caption.Text"=w318) -> ()  [unwired: 2 in, 2 out]
          }
          frame "Compressor", "Digital Out" {
            w326 = FALSE ("Visible")
            # "Get direction and finish"
            n187 = property on="Motor" class="Clust (strict)"("Visible"=w326) -> ()  [unwired: 2 in, 2 out]
            n188 = property on="Test Slider" class="Slide (strict)"("Visible"=w326) -> ()  [unwired: 2 in, 2 out]
            n189 = property on="Test Ring" class="Ring (strict)"("Visible"=w326) -> ()  [unwired: 2 in, 2 out]
            n190 = property on="On/Off" class="Bool (strict)"("Visible"=TRUE, "Caption.Text"=w327) -> ()  [unwired: 2 in, 2 out]
            n191 = property on="Rev/Fwd" class="Clust (strict)"("Visible"=FALSE) -> ()  [unwired: 2 in, 2 out]
          }
          frame "Camera" {
            n192 = call <vilib>:"Get Last Path Segment.vi"("String in"=w334) -> ("String out"=w335:string)  [unwired: 10 in]
            n193 = property on="On/Off" class="Bool (strict)"("Visible"=FALSE) -> ()  [unwired: 2 in, 2 out]
            n194 = property on="Motor" class="Clust (strict)"("Visible"=FALSE) -> ()  [unwired: 2 in, 2 out]
            n195 = property on="Rev/Fwd" class="Clust (strict)"("Visible"=FALSE) -> ()  [unwired: 2 in, 2 out]
            n196 = case shown="\"White Balance  **\"" w335 {
              tunnel: w334 -> [w341 w350 w359 w368 w377 _ w383]
              tunnel: w333 -> [w339 w347 w356 w365 w374 _ _]
              frame "Size  **" {
                n197 = Index Array(array=w339) -> (element=w338:cluster{string[]})  [unwired: 1 in]
                n198 = call <vilib>:"NT Read String.vi"("Name"=w341) -> ("String"=w340:string)  [unwired: 9 in, 1 out]
                n199 = Unbundle(w338) -> (w336:string[])
                n200 = Match First String(2:w336, 3:w340) -> (0:w337:i32)  [unwired: 1 out]
                n201 = property on="Test Ring" class="Ring (strict)"("Value"=w337, "Strings []"=w336) -> ()  [unwired: 2 in, 2 out]
                n202 = property on="Test Ring" class="Ring (strict)"("Visible"=TRUE) -> ()  [unwired: 2 in, 2 out]
                n203 = property on="Test Slider" class="Slide (strict)"("Visible"=FALSE) -> ()  [unwired: 2 in, 2 out]
              }
              frame "White Balance  **" {
                n204 = Index Array(array=w347, index=1) -> (element=w348:cluster{string[]})
                n205 = call <vilib>:"NT Read String.vi"("Name"=w350) -> ("String"=w349:string)  [unwired: 9 in, 1 out]
                n206 = Unbundle(w348) -> (w345:string[])
                n207 = Match First String(2:w345, 3:w349) -> (0:w344:i32)  [unwired: 1 out]
                n208 = property on="Test Ring" class="Ring (strict)"("Value"=w344, "Strings []"=w345) -> ()  [unwired: 2 in, 2 out]
                n209 = property on="Test Ring" class="Ring (strict)"("Visible"=TRUE) -> ()  [unwired: 2 in, 2 out]
                n210 = property on="Test Slider" class="Slide (strict)"("Visible"=FALSE) -> ()  [unwired: 2 in, 2 out]
              }
              frame "Exposure  **" {
                n211 = Index Array(array=w356, index=2) -> (element=w357:cluster{string[]})
                n212 = call <vilib>:"NT Read String.vi"("Name"=w359) -> ("String"=w358:string)  [unwired: 9 in, 1 out]
                n213 = Unbundle(w357) -> (w353:string[])
                n214 = Match First String(2:w353, 3:w358) -> (0:w354:i32)  [unwired: 1 out]
                n215 = property on="Test Ring" class="Ring (strict)"("Value"=w354, "Strings []"=w353) -> ()  [unwired: 2 in, 2 out]
                n216 = property on="Test Ring" class="Ring (strict)"("Visible"=TRUE) -> ()  [unwired: 2 in, 2 out]
                n217 = property on="Test Slider" class="Slide (strict)"("Visible"=FALSE) -> ()  [unwired: 2 in, 2 out]
              }
              frame "Exposure Priority  **" {
                n218 = Index Array(array=w365, index=3) -> (element=w366:cluster{string[]})
                n219 = call <vilib>:"NT Read String.vi"("Name"=w368) -> ("String"=w367:string)  [unwired: 9 in, 1 out]
                n220 = Unbundle(w366) -> (w362:string[])
                n221 = Match First String(2:w362, 3:w367) -> (0:w363:i32)  [unwired: 1 out]
                n222 = property on="Test Ring" class="Ring (strict)"("Value"=w363, "Strings []"=w362) -> ()  [unwired: 2 in, 2 out]
                n223 = property on="Test Ring" class="Ring (strict)"("Visible"=TRUE) -> ()  [unwired: 2 in, 2 out]
                n224 = property on="Test Slider" class="Slide (strict)"("Visible"=FALSE) -> ()  [unwired: 2 in, 2 out]
              }
              frame "Color Enable  **" {
                n225 = Index Array(array=w374, index=4) -> (element=w375:cluster{string[]})
                n226 = call <vilib>:"NT Read String.vi"("Name"=w377) -> ("String"=w376:string)  [unwired: 9 in, 1 out]
                n227 = Unbundle(w375) -> (w371:string[])
                n228 = Match First String(2:w371, 3:w376) -> (0:w372:i32)  [unwired: 1 out]
                n229 = property on="Test Ring" class="Ring (strict)"("Value"=w372, "Strings []"=w371) -> ()  [unwired: 2 in, 2 out]
                n230 = property on="Test Ring" class="Ring (strict)"("Visible"=TRUE) -> ()  [unwired: 2 in, 2 out]
                n231 = property on="Test Slider" class="Slide (strict)"("Visible"=FALSE) -> ()  [unwired: 2 in, 2 out]
              }
              frame Default {
                n232 = property on="Test Ring" class="Ring (strict)"("Visible"=FALSE) -> ()  [unwired: 2 in, 2 out]
                n233 = property on="Test Slider" class="Slide (strict)"("Visible"=FALSE) -> ()  [unwired: 2 in, 2 out]
              }
              frame "Brightness  **", "Color Level  **", "Compression  **", "FPS  **", "Sharpness  **" {
                n234 = call <vilib>:"NT Read Number.vi"("Name"=w383) -> ("Numeric"=w382:dbl)  [unwired: 9 in, 1 out]
                n235 = local write "Test Slider"(w382) -> ()
                n236 = property on="Test Slider" class="Slide (strict)"("Visible"=TRUE, "Scale.Maximum"=100.0 ("Scale.Range:Maximum")) -> ()  [unwired: 2 in, 2 out]
                n237 = property on="Test Ring" class="Ring (strict)"("Visible"=FALSE) -> ()  [unwired: 2 in, 2 out]
              }
            }
          }
        }
        n238 = property on="Progress" class="Clust (strict)"("Visible"=FALSE) -> ()  [unwired: 2 in, 2 out]
      }
      event "Test Name": Mouse Enter {
        # "Populate the ring with the list of tests"
        n239 = event-data() -> ()  [unwired: 1 in, 1 out]
        n240 = call <vilib>:"NT Read String Array.vi"("Name"="TestMode/TestList") -> ("String Array"=w391:string[])  [unwired: 9 in, 1 out]
        n241 = Build Array (concatenate)("Select the test to run...", w391) -> (w390:string[])
        n242 = property on="Test Name" class="Ring (strict)"("Strings []"=w390) -> ()  [unwired: 2 in, 2 out]
      }
      event "Test Name": Value Change {
        w393 = FALSE ("Visible")
        # "Tell the robot the test name to run"
        n243 = event-data() -> ("NewVal"=w397:u16)  [unwired: 1 in]
        n244 = property on="Test Name" class="Ring (strict)"() -> ("Strings []"=w398:string[])  [unwired: 2 in, 2 out]
        n245 = local write "Progress"(T6 {"Test Progress"=0, "Test Progress Text"=""} ("Progress")) -> ()
        n246 = Index Array(array=w398, index=w397) -> (element=w396:string)
        n247 = call <vilib>:"NT Write String.vi"("String"=w396, "Name"="TestMode/TestName") -> ()  [unwired: 9 in, 1 out]
        n248 = property on="Progress" class="Clust (strict)"("Visible"=TRUE) -> ()  [unwired: 2 in, 2 out]
        n249 = property on="Motor" class="Clust (strict)"("Visible"=w393) -> ()  [unwired: 2 in, 2 out]
        n250 = property on="Test Slider" class="Slide (strict)"("Visible"=w393) -> ()  [unwired: 2 in, 2 out]
        n251 = property on="On/Off" class="Bool (strict)"("Visible"=w393) -> ()  [unwired: 2 in, 2 out]
        n252 = property on="Rev/Fwd" class="Clust (strict)"("Visible"=w393) -> ()  [unwired: 2 in, 2 out]
        n253 = property on="Test Ring" class="Ring (strict)"("Visible"=w393) -> ()  [unwired: 2 in, 2 out]
      }
      event Mouse Enter {
        # "Populate the combo box with the list of autonomous options"
        n254 = event-data() -> ()  [unwired: 1 in, 1 out]
        n255 = call <vilib>:"NT Read String Array.vi"("Name"="Auto List") -> ("String Array"=w400:string[])  [unwired: 9 in, 1 out]
        n256 = property on="Select Auto" class="CmbBox (strict)"("Strings[]"=w400) -> ()  [unwired: 2 in, 2 out]
      }
      event Value Change {
        # "User modified the Auto Selection. Write to NT variable so robot knows."
        n257 = event-data() -> ("NewVal"=w403:T1)  [unwired: 1 in]
        n258 = call <vilib>:"NT Write String.vi"("String"=w403, "Name"="Auto Selector") -> ()  [unwired: 9 in, 1 out]
      }
      event "Command Selection": Value Change {
        # "Get the params and show in table"
        n259 = event-data() -> ("NewVal"=w409:i32)  [unwired: 1 in]
        n260 = property on="Command Selection" class="MCListbox (strict)"() -> ("ItemNames"=w407:string[][])  [unwired: 2 in, 2 out]
        n261 = call <vilib>:"WPI_DashboardUpdate Command Params.vi"("NewVal"=w409, "Commands"=w407, "Param Tbl"=w408) -> ()  [unwired: 8 in, 1 out]
      }
      event "Execute Command": Value Change {
        # "Started one, Unique ID holds\nresponse"
        n262 = event-data() -> ()  [unwired: 1 in, 1 out]
        n263 = property on="Command Selection" class="MCListbox (strict)"() -> ("ItemNames"=w420:string[][])  [unwired: 2 in, 2 out]
        n264 = Index Array(array=w420, index (row)="Command Selection", index (col)=0) -> (element=w418:string)
        n265 = call <vilib>:"Invoke Commands.vi"("Command Params"="Command Params", "Function Name"=w418) -> ("Params"=w414:u8, "Started"=w413:bool)  [unwired: 7 in, 1 out]
        n266 = Array Subset(array="Command Params", length (row)=w414) -> (w415:string[][])  [unwired: 3 in]
        n267 = Select(t="Executing" ("Cmd Status"), s=w413, f="" ("Cmd Status")) -> (s? t:f=→"Cmd Status":string)
      }
      event "Command Selection": Double Click {
        n268 = event-data() -> ("Row"=w428:i32)  [unwired: 1 in]
        n269 = property on="Command Selection" class="MCListbox (strict)"() -> ("ItemNames"=w431:string[][])  [unwired: 2 in, 2 out]
        n270 = local read "Command Params"() -> (w427:string[][])
        n271 = Index Array(array=w431, index (row)=w428, index (col)=0) -> (element=w429:string)
        n272 = call <vilib>:"Invoke Commands.vi"("Command Params"=w427, "Function Name"=w429) -> ("Params"=w426:u8, "Started"=w421:bool)  [unwired: 7 in, 1 out]
        n273 = Array Subset(array=w427, length (row)=w426) -> (w425:string[][])  [unwired: 3 in]
        n274 = Select(t="Executing" ("Cmd Status"), s=w421, f="" ("Cmd Status")) -> (s? t:f=w422:string)
        n275 = local write "Cmd Status"(w422) -> ()
      }
      event "CheckList": Double Click {
        # "Shift clears all"
        # "Update symbols on the listbox"
        n276 = event-data() -> ("PlatMods.Shift"=w433:bool, "Row"=w435:i32)  [unwired: 1 in]
        n277 = case shown="True" w433 {
          tunnel: w435 -> [w439 _]
          tunnel: 1 -> [w438 _]
          frame False {
            n278 = property on="CheckList" class="LstBox (strict)"() -> ("Item Symbols"=w437:i32[])  [unwired: 2 in, 2 out]
            n279 = Replace Array Subset(array=w437, new element=w438, index=w439) -> (w436:i32[])
            n280 = property on="CheckList" class="LstBox (strict)"("Item Symbols"=w436) -> ()  [unwired: 2 in, 2 out]
          }
          frame True {
            w440 = 0 ("Top Row")
            n281 = property on="CheckList" class="LstBox (strict)"() -> ("Number of Rows"=w442:u32)  [unwired: 2 in, 2 out]
            n282 = Initialize Array(0, w442) -> (w441:i32[])
            n283 = property on="CheckList" class="LstBox (strict)"("Top Row"=w440, "Value"=w440, "Item Symbols"=w441) -> ()  [unwired: 2 in, 2 out]
          }
        }
      }
      event "CheckList": Key Down {
        # "Update symbols on the listbox\nLeft and right keys check and uncheck"
        n284 = event-data() -> ("VKey"=w446:T20)  [unwired: 1 in]
        n285 = case shown="\"Left\", \"Right\"" w446 {
          selector: w446 -> [w451 _]
          tunnel: eventvkey."Left" ("VKey") -> [w449 _]
          frame "Left", "Right" {
            n286 = Equal?(x=w449, y=w451) -> (x = y?=w450:bool)
            n287 = Select(t=0, s=w450, f=1) -> (s? t:f=w452:i32)
            n288 = property on="CheckList" class="LstBox (strict)"() -> ("Item Symbols"=w455:i32[])  [unwired: 2 in, 2 out]
            n289 = Replace Array Subset(array=w455, new element=w452, index="CheckList") -> (w454:i32[])
            n290 = property on="CheckList" class="LstBox (strict)"("Item Symbols"=w454) -> ()  [unwired: 2 in, 2 out]
          }
          frame Default {
          }
        }
      }
      event "Motor.Enable": Value Change {
        # "When the test mode otor enable helper is set, update that\ntree row item's value"
        n291 = event-data() -> ("NewVal"=w461:bool)  [unwired: 1 in]
        n292 = Unbundle("Motor") -> ("Value"=w460:dbl)  [unwired: 1 out]
        n293 = Select(t=w460, s=w461, f=0.0) -> (s? t:f=w458:dbl)
        n294 = call <vilib>:"NT Write Number.vi"("Numeric"=w458, "Name"=w457) -> ()  [unwired: 9 in, 1 out]
      }
      event "Test Slider": Value Change {
        # "When the test mode slider helper is set, update that\ntree row item's value"
        n295 = event-data() -> ("NewVal"=w464:dbl)  [unwired: 1 in]
        n296 = call <vilib>:"NT Write Number.vi"("Numeric"=w464, "Name"=w465) -> ()  [unwired: 9 in, 1 out]
      }
      event "On/Off": Value Change {
        # "When the test mode on/off helper value is set, update that\ntree row item's value"
        n297 = event-data() -> ("NewVal"=w469:bool)  [unwired: 1 in]
        n298 = Boolean To (0,1)(Boolean=w469) -> (0, 1=w468:i16)
        n299 = call <vilib>:"NT Write Number.vi"("Numeric"=w468, "Name"=w467) -> ()  [unwired: 9 in, 1 out]
      }
      event "Rev/Fwd": Value Change {
        # "When the test mode helper value for relays is set, update that\ntree row item's value"
        n300 = event-data() -> ("NewVal.Forward"=w477:bool, "NewVal.Reverse"=w476:bool)  [unwired: 1 in]
        n301 = Boolean To (0,1)(Boolean=w477) -> (0, 1=w473:i16)
        n302 = Boolean To (0,1)(Boolean=w476) -> (0, 1=w475:i16)
        n303 = Negate(x=w475) -> (-x=w474:i16)
        n304 = Add(x=w473, y=w474) -> (x+y=w472:i16)
        n305 = call <vilib>:"NT Write Number.vi"("Numeric"=w472, "Name"=w471) -> ()  [unwired: 9 in, 1 out]
      }
      event "Test Ring": Value Change {
        # "When a test mode helper value is selected from the ring,\nset the tree item's variable to the string value"
        n306 = event-data() -> ("NewVal"=w481:u16)  [unwired: 1 in]
        n307 = property on="Test Ring" class="Ring (strict)"() -> ("Strings []"=w482:string[])  [unwired: 2 in, 2 out]
        n308 = Index Array(array=w482, index=w481) -> (element=w480:string)
        n309 = call <vilib>:"NT Write String.vi"("String"=w480, "Name"=w479) -> ()  [unwired: 9 in, 1 out]
      }
      event "Rec Mode": Value Change {
        # "Update globals for recording mode and path to read log from.\nClear when logging and let NetworkTables set path for vision to\nuse."
        n310 = event-data() -> ("NewVal"=w493:enum32{"Stop", "Record", "Playback"})  [unwired: 1 in]
        n311 = global write "WPI_DashboardLogging Global.vi" "Logging Filename"(path "") -> ()
        n312 = global write "WPI_DashboardLogging Global.vi" "Recording"(w493) -> ()
        n313 = case shown="\"Playback\"" w493 {
          tunnel: w492 -> [_ w495 w504]
          tunnel: [_ _ w503] -> w490
          tunnel: [_ _ w502] -> _
          tunnel: w488 -> [_ _ w500]
          tunnel: cluster{i32, i32} {-250, 170} -> [_ _ w499]
          tunnel: [_ _ T21 {"Image Size"=TRUE, "Image Type"=TRUE, "Pixel Value"=TRUE, "ROI Information"=TRUE, "Zoom Factor"=FALSE} ("Image Information Shown:All Elements")] -> w483
          tunnel: [_ _ TRUE ("Zoom Factor")] -> w484
          tunnel: w486 -> [_ _ w496]
          frame Default {
          }
          frame "Stop", "Record" {
            # "Place Window too"
            n314 = invoke class="VI" method="FP.Close"(reference=w495) -> (reference out=w494:refnum<vi>)  [unwired: 2 in, 2 out]
            n315 = invoke class="VI" method="Abort VI"(reference=w494) -> ()  [unwired: 2 in, 3 out]
          }
          frame "Playback" {
            n316 = call "Open Playback Panel.vi"("Offset"=w499, "DB VI Ref"=w500, "Playback in"=w504) -> ("Playback out"=w501:refnum<vi>)  [unwired: 8 in]
            n317 = register-events(w501, w496) -> (reference out=w503:refnum<event-registration>, error out=w502:errorcluster)  [unwired: 2 in]
          }
        }
        n318 = property on="Camera Image Right" class="ImageControl"("Image Information Shown"=w483, "Image Information Visible"=w484) -> ()  [unwired: 2 in, 2 out]
        n319 = property on="Camera Image" class="ImageControl"("Image Information Shown"=w483, "Image Information Visible"=w484) -> ()  [unwired: 2 in, 2 out]
        n320 = call <vilib>:"WPI_DashboardNT Log FieldName Cache.vi"("Operation"=enum16{"Lookup/Add", "Index", "Clear"}."Clear") -> ()  [unwired: 8 in, 3 out]
      }
      event Panel Close {
        w506 = enum32{"Stop", "Record", "Playback"}."Stop" ("Rec Mode")
        # "Playback window has been closed, abort"
        n321 = event-data() -> ()  [unwired: 1 in, 4 out]
        n322 = local write "Rec Mode"(w506) -> ()
        n323 = global write "WPI_DashboardLogging Global.vi" "Recording"(w506) -> ()
      }
      event Panel Close {
        # "Abort playback window and ourself"
        n324 = event-data() -> ()  [unwired: 1 in, 4 out]
        n325 = invoke class="VI" method="FP.Close"(reference=w510) -> (reference out=w509:refnum<vi>)  [unwired: 2 in, 2 out]
        n326 = invoke class="VI" method="Abort VI"(reference=w509) -> (error out=w508:errorcluster)  [unwired: 2 in, 2 out]
        n327 = invoke class="VI" method="Abort VI"(error in=w508) -> ()  [unwired: 2 in, 3 out]
      }
      event User Event {
        n328 = event-data() -> ("IDs"=w517:cluster{"RPC field ID":u16, "Unique ID":u16}, "String"=w516:string)  [unwired: 1 in]
        n329 = Bundle("IDs"=w517, "String"=w516) -> (w515:T10)  [unwired: 1 in]
        n330 = call <vilib>:"Retrieve RPC Response.vi"("RPC Response"=w515) -> ("Output"=w513:string[][])  [unwired: 10 in]
        n331 = Build Array (concatenate)(w511, w513) -> (w512:string[][])
        n332 = local write "Command Params"(w512) -> ()
        n333 = local write "Cmd Status"("" ("Cmd Status")) -> ()
      }
      event "Tree": Double Click {
        n334 = event-data() -> ("PlatMods"=w523:T24, "Tag"=w520:string)  [unwired: 1 in]
        n335 = Unbundle(w523) -> ("Shift"=w522:bool)  [unwired: 4 out]
        n336 = String Subset(string=w520, length (rest)=1 ("length (rest)")) -> (substring=w519:string)  [unwired: 1 in]
        n337 = Not(x=w522) -> (.not. x?=w521:bool)
        n338 = case shown="\"/\"" w519 {
          tunnel: w520 -> [_ w526]
          tunnel: w521 -> [_ w525]
          frame Default {
          }
          frame "/" {
            n339 = call <vilib>:"NT Update Persistence.vi"("Persistence"=w525, "Name"=w526) -> ()  [unwired: 9 in, 1 out]
          }
        }
      }
    }
  }
  n340 = while {
    tunnel: w63 -> [w528]
    i -> [w531]
    stop <- FALSE stop-if-true
    n341 = Wait (ms)(milliseconds to wait=u32 100) -> ()  [unwired: 1 out]
    n342 = case shown="\"Playback\"" "Rec Mode" {
      tunnel: w531 -> [_ _ w546]
      tunnel: [u32 2829099 ("Base Color") u32 11141120 ("Target Color") w535] -> w527
      frame "Stop", Default {
        # "Reset the color, extra updates don't cost much"
      }
      frame "Record" {
      }
      frame "Playback" {
        # "Playback"
        n343 = Quotient & Remainder(x=w546, y=u32 50 ("milliseconds to wait")) -> (x-y*floor(x/y)=w542:u32)  [unwired: 1 out]
        n344 = Divide(x=w542, y=u32 50 ("milliseconds to wait")) -> (x/y=w539:dbl)
        n345 = Multiply(x=6.283185307179586, y=w539) -> (x*y=w544:dbl)
        n346 = Sine(x=w544) -> (sin(x)=w543:dbl)
        n347 = Absolute Value(x=w543) -> (abs(x)=w536:dbl)
        n348 = call "Interpolate RGB Color.vi"("Proportion"=w536, "Target Color"=u32 30976, "Base Color"=u32 2829099) -> ("Result Color"=w535:u32)  [unwired: 8 in]
      }
    }
    n349 = property class="Pane"(reference=w528, "PaneColor"=w527) -> ()  [unwired: 1 in, 2 out]
  }
  n350 = local write "Dashboard Tab"(T3."Drive" ("Dashboard Tab")) -> ()
  n351 = property on="On/Off" class="Bool (strict)"("Visible"=w34) -> ()  [unwired: 2 in, 2 out]
  n352 = property on="Motor" class="Clust (strict)"("Visible"=w34) -> ()  [unwired: 2 in, 2 out]
  n353 = property on="Progress" class="Clust (strict)"("Visible"=w34) -> ()  [unwired: 2 in, 2 out]
  n354 = property on="Test Ring" class="Ring (strict)"("Visible"=w34) -> ()  [unwired: 2 in, 2 out]
  n355 = property on="Rev/Fwd" class="Clust (strict)"("Visible"=w34) -> ()  [unwired: 2 in, 2 out]
  n356 = local write "Command Selection"(u16 0 ("milliseconds to wait")) -> ()
  n357 = while {
    tunnel: u16 1741 ("timeout ms (25000)") -> [w548]
    stop <- FALSE stop-if-true
    n358 = TCP Create Listener(10:w548) -> (0:w547:errorcluster, 3:w549:refnum<k5>)  [unwired: 4 in, 1 out]
    n359 = case shown="No Error" w547 {
      selector: w547 -> [w551 _]
      tunnel: w549 -> [w552 _]
      frame No Error {
        n360 = while {
          tunnel: w552 -> [w555]
          tunnel: w551 -> [w554]
          stop <- FALSE stop-if-true
          n361 = TCP Wait On Listener(8:w554, 11:w555) -> (0:w556:errorcluster, 4:w557:refnum<k5>)  [unwired: 2 in, 3 out]
          n362 = local write "TCP"(w557) -> ()
          n363 = case shown="No Error" w556 {
            frame No Error {
            }
            frame Error {
              n364 = Wait (ms)(milliseconds to wait=u32 1000) -> ()  [unwired: 1 out]
            }
          }
        }
      }
      frame Error {
        n365 = Wait (ms)(milliseconds to wait=u32 1000) -> ()  [unwired: 1 out]
      }
    }
  }
  n366 = local write "Command Params"(string[][] [] ("Command Params")) -> ()
  n367 = global write "WPI_DashboardLogging Global.vi" "Recording"(w57) -> ()
  n368 = local write "Rec Mode"(w57) -> ()
